vi "pra_globalnord.vi"() -> ()   [LabVIEW 2018]
panel:
  out "ブール":bool
  out "ブール 2":bool
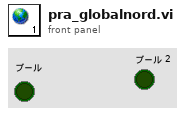
[diagram p1: front panel]
diagram:
